vi "Reference.vi"(8 "error in (no error)":errorcluster, 10 "Instrument":refnum<class>, 11 "InstrPtr in":refnum<class "InstrPtr.lvclass">) -> (0 "error out":errorcluster)   [LabVIEW 2017, in "InstrPtr.lvclass"]
doc: "Reference: \"checks in\" the object instance and unlocks it so other threads / processes can use it."
uses:
  InstrPtr.lvclass
  InstrPtr.lvclass/InstrPtr.ctl
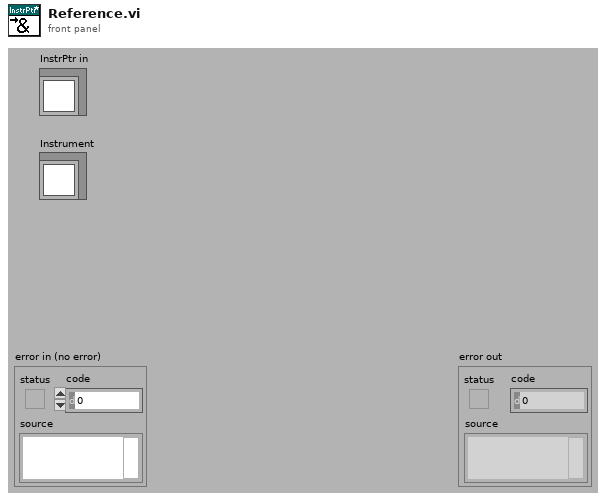
[diagram p1: front panel]
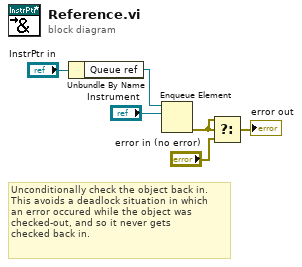
[diagram p0: block diagram]
diagram:
  # "Unconditionally check the object back in.\nThis avoids a deadlock situation in which\nan error occured while the object was\nchecked-out, and so it never gets\nchecked back in."
  n1 = Unbundle By Name("InstrPtr in") -> ("Queue ref"=w4:refnum<queue>)
  n2 = Enqueue Element(queue=w4, element="Instrument") -> (error out=w3:errorcluster)  [unwired: 1 in, 3 out]
  n3 = Select(t=w3, s=w3, f="error in (no error)") -> (s? t:f=→"error out":errorcluster)
